vi "Parse FSN.vi"(8 "error in (no error)":errorcluster, 11 "FSN in":string) -> (0 "error out":errorcluster, 3 "FSN out":u8)   [LabVIEW 2018, in "Config Parser BML.lvlib" / "Config Parser BML.lvclass"]
uses:
  Config Parser BML.lvclass
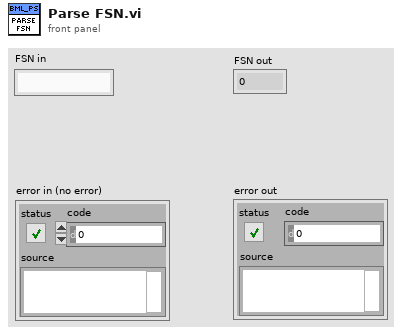
[diagram p1: front panel]
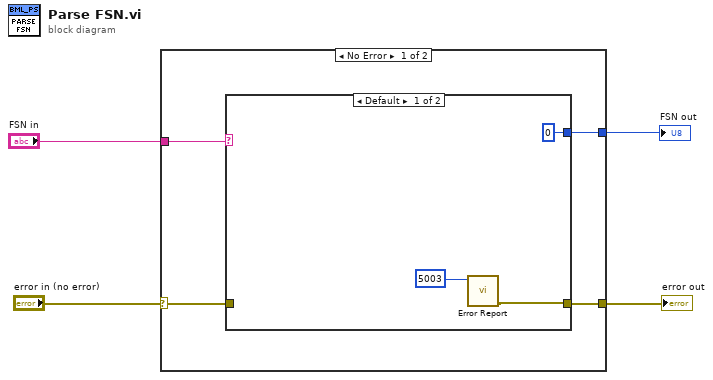
[diagram p0: block diagram]
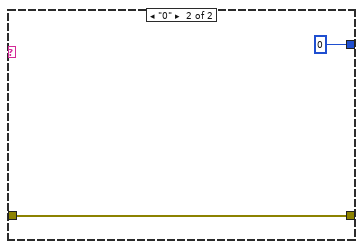
[diagram p2: hidden frame]
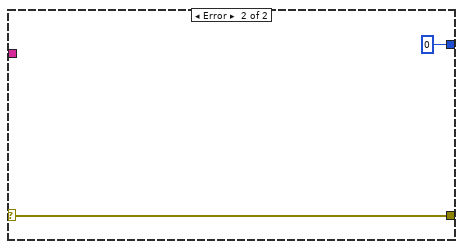
[diagram p3: hidden frame]
diagram:
  n1 = case shown="No Error" "error in (no error)" {
    selector: "error in (no error)" -> [w6 w15]
    tunnel: "FSN in" -> [w8 _]
    tunnel: [w5 w15] -> w2
    tunnel: [w7 u8 0 ("FSN out")] -> w1
    frame No Error {
      n2 = case shown="Default" w8 {
        tunnel: [u8 0 ("FSN out") u8 0 ("FSN out")] -> w7
        tunnel: w6 -> [_ w12]
        tunnel: [w10 w12] -> w5
        frame Default {
          n3 = call "Error Report.vi"("Error Code"=i16 5003) -> ("error out"=w10:errorcluster)  [unwired: 10 in]
        }
        frame "0" {
        }
      }
    }
    frame Error {
    }
  }
  "error out" <- w2
  "FSN out" <- w1
